vi "CurrentAllServoData.vi"(8 "New All Servo Data":T1 {"status"."position" min=0 max=180 step=1}, 11 "Operation":T3) -> (3 "Current All Servo Data":T1 {"status"."position" min=0 max=180 step=1})   [LabVIEW 2024]
uses:
  DataTypes/AllServoData.ctl
  DataTypes/ServoStatus.ctl
  DataTypes/OperationTypeForFunctionalGlobalVariable.ctl
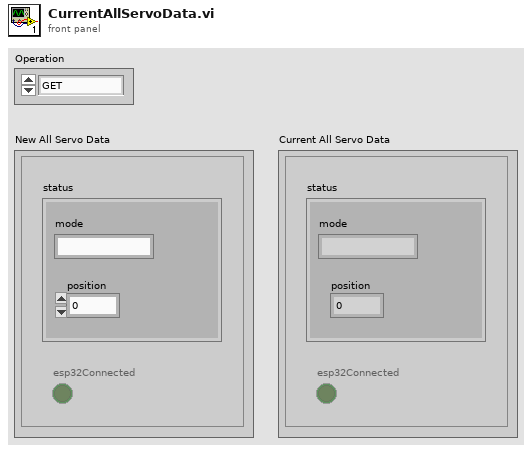
[diagram p1: front panel]
types:
  T1 = typedef "AllServoData.ctl" = cluster{"status":T2, "esp32Connected":bool}
  T2 = typedef "ServoStatus.ctl" = cluster{"mode":string, "position":i16}
  T3 = typedef "OperationTypeForFunctionalGlobalVariable.ctl" = enum16{"GET", "SET"}
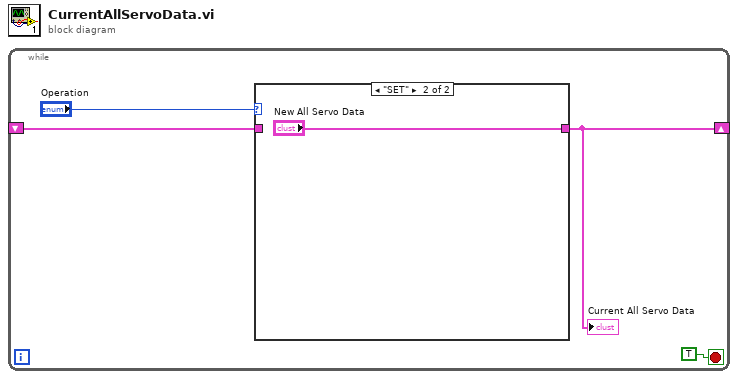
[diagram p0: block diagram]
diagram:
  n1 = while {
    shift-right: [w1] -> _
    shift-left: _ -> [w2]
    stop <- TRUE stop-if-true
    n2 = case shown="\"SET\"" "Operation" {
      tunnel: w2 -> [w5 _]
      tunnel: [w5 "New All Servo Data"] -> w1
      frame "GET", Default {
      }
      frame "SET" {
      }
    }
    "Current All Servo Data" <- w1
  }
